vi "test Read Custom TagDistanceArray.vi"(8 "error in (no error)":errorcluster, 11 "TestCase in":refnum<class "AnchorTests.lvclass">) -> (0 "error out":errorcluster, 3 "TestCase out":refnum<class "AnchorTests.lvclass">)   [LabVIEW 2014, in "AnchorTests.lvclass"]
uses:
  AnchorTests.lvclass
  SPLAT/Anchor/Anchor.lvclass
  <vilib>/addons/_JKI Toolkits/VI Tester/TestCase.llb/TestCase.lvclass
  SPLAT/Tag.lvclass
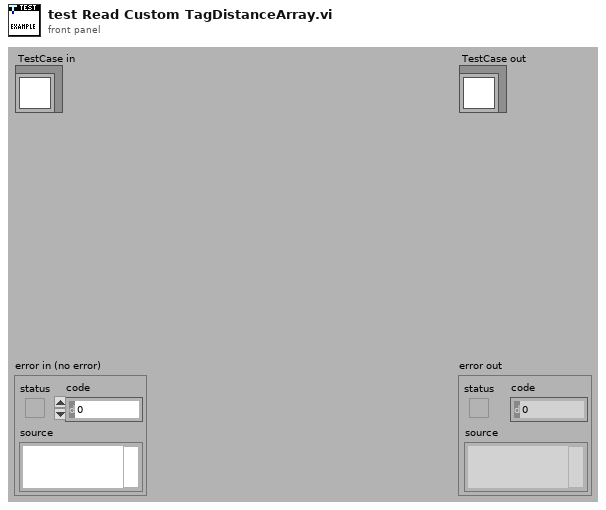
[diagram p1: front panel]
types:
  T1 = cluster{"Tag Out":refnum<class "Tag.lvclass">, "Distance":dbl}
  T2 = cluster{"Tag Out":refnum<class "Tag.lvclass">, "Distance":dbl}[]
  T3 = cluster{"Tag.lvclass":refnum<class "Tag.lvclass">, "Distance":dbl}[]
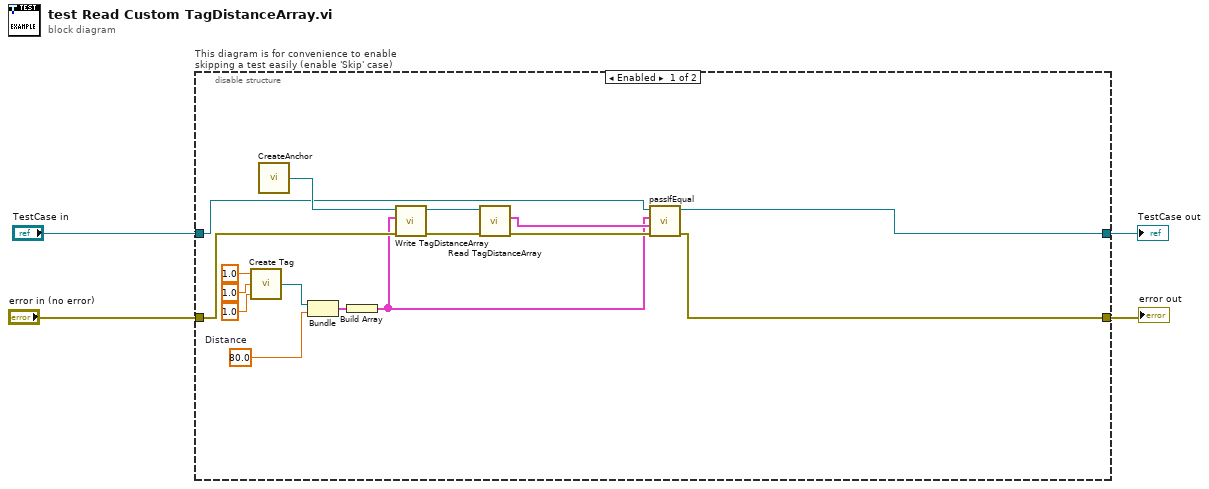
[diagram p0: block diagram]
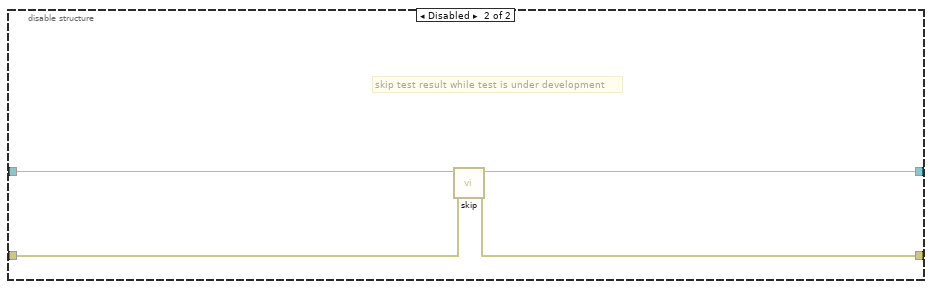
[diagram p2: hidden frame]
diagram:
  n1 = disable-structure "This diagram is for convenience to enable skipping a test easily (enable 'Skip' case)" shown="Enabled" {
    disable-tunnel: "TestCase in" -> [w7 w24]
    disable-tunnel: [w5 w22] -> w1
    disable-tunnel: [w6 w23] -> w3
    disable-tunnel: "error in (no error)" -> [w13 w21]
    frame Enabled {
      w15 = 80.0  # Distance
      n2 = call "Create Tag.vi"("TagY"=1.0, "TagX"=1.0, "TagID"=1.0) -> ("Tag Out"=w16:refnum<class "Tag.lvclass">)
      n3 = call "CreateAnchor.vi"() -> ("Anchor Out"=w20:refnum<class "Anchor.lvclass">)  [unwired: 3 in]
      n4 = Bundle("Tag Out"=w16, "Distance"=w15) -> (w14:T1)  [unwired: 1 in]
      n5 = Build Array(w14) -> (w8:T2)
      n6 = call-dynamic "Write TagDistanceArray.vi"("error in (no error)"=w13, "TagDistanceArray"=w8, "Anchor in"=w20) -> ("error out"=w12:errorcluster, "Anchor out"=w11:refnum<class "Anchor.lvclass">)  [unwired: 7 in]
      n7 = call-dynamic "Read TagDistanceArray.vi"("error in (no error)"=w12, "Anchor in"=w11) -> ("error out"=w10:errorcluster, "TagDistanceArray"=w9:T3)  [unwired: 7 in, 1 out]
      n8 = call-dynamic "passIfEqual.vi"("error in (no error)"=w10, "y"=w9, "x"=w8, "TestCase in"=w7) -> ("error out"=w6:errorcluster, "TestCase out"=w5:refnum<class "AnchorTests.lvclass">)  [unwired: 6 in]
    }
    frame Disabled {
      # "skip test result while test is under development"
      n9 = call <vilib>:"skip.vi"("error in (no error)"=w21, "TestCase in"=w24) -> ("error out"=w23:errorcluster, "TestCase out"=w22:refnum<class "AnchorTests.lvclass">)  [unwired: 8 in]
    }
  }
  "error out" <- w3
  "TestCase out" <- w1
